vi "timestamp before 1904.vi"() -> ()   [LabVIEW 2019]
panel:
  out "time stamp":timestamp
  out "Error Out":errorcluster
  in  "TDMS File":path=path "C:/Python/projects/nitdms/tests/tdms_files/timestamp before 1904.tdms"
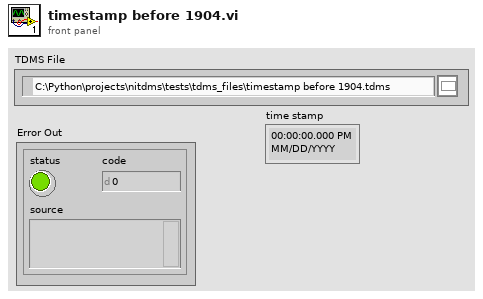
[diagram p1: front panel]
types:
  T1 = enum16{"open", "open or create", "create or replace", "create", "open (read-only)"}
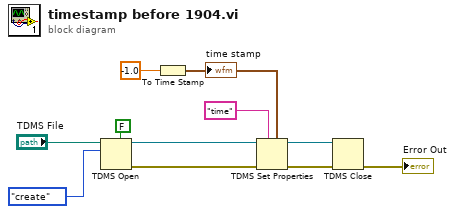
[diagram p0: block diagram]
diagram:
  n1 = TDMS Open(5:FALSE ("create index file? (T)"), 10:T1."create" ("operation (0:open)"), 11:"TDMS File") -> (0:w7:errorcluster, 3:w6:refnum<k34>)  [unwired: 4 in]
  n2 = To Time Stamp(1:-1.0) -> (0:w1:timestamp)
  "time stamp" <- w1
  n3 = TDMS Set Properties(5:w1, 7:"time", 8:w7, 11:w6) -> (0:w5:errorcluster, 3:w4:refnum<k34>)  [unwired: 2 in, 2 out]
  n4 = TDMS Close(8:w5, 11:w4) -> (0:→"Error Out":errorcluster)  [unwired: 1 out]
